vi "libssh2_channel_open_session.vi"(5 "packet_size (32 KiB)":u32=32768, 7 "window_size (2 MiB)":u32=2097152, 8 "error in (no error)":errorcluster, 11 "session":T1) -> (0 "error out":errorcluster, 3 "channel":T2)   [LabVIEW 2013, in "libssh2.lvlib"]
doc: "Establishes a new channel."
uses:
  libssh2.lvlib
  Channel Refnum.ctl
  Session Refnum.ctl
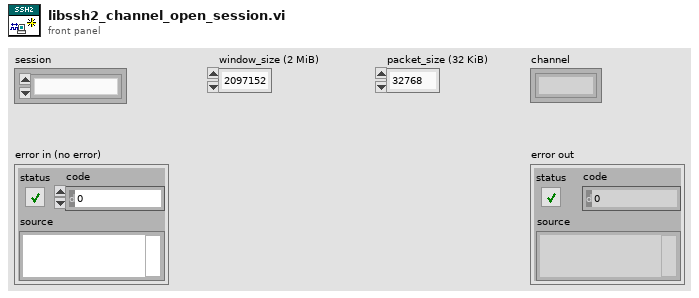
[diagram p1: front panel]
types:
  T1 = typedef "libssh2.lvlib/Session Refnum.ctl" = refnum<k1>
  T2 = typedef "libssh2.lvlib/Channel Refnum.ctl" = refnum<k1>
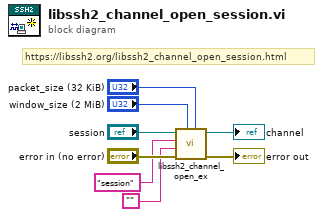
[diagram p0: block diagram]
diagram:
  # "https://libssh2.org/libssh2_channel_open_session.html"
  n1 = call "libssh2_channel_open_ex.vi"("packet_size (32 KiB)"="packet_size (32 KiB)", "window_size (2 MiB)"="window_size (2 MiB)", "error in (no error)"="error in (no error)", "message"="", "channel_type"="session", "session"="session") -> ("error out"=→"error out":errorcluster, "channel"=→"channel":T2)  [unwired: 4 in]
